vi "Logging Message Loop.vi"(8 "error in (no error)":errorcluster, 10 "Data Queue":T1, 11 "Message Queues":T2) -> (0 "error out":errorcluster)   [LabVIEW 2021, in "IMU Logging.lvlib"]
doc: "The message loop subVI to handle messages pertaining to logging data."
uses:
  IMU Logging.lvlib
  support/Message Queue/All Message Queues.ctl
  support/Message Queue/Message Cluster.ctl
  Acquisition/IMU Data Queue.ctl
  IMU TimeDataStruct.ctl
  Logging Configuration.ctl
  Logging State.ctl
  support/Message Queue/Enqueue Message (Single).vi
  <vilib>/Utility/error.llb/Error Cluster From Error Code.vi
  <vilib>/ErrorRing/Error Ring.xnode
  support/Message Queue/IMU Message Queue.lvlib
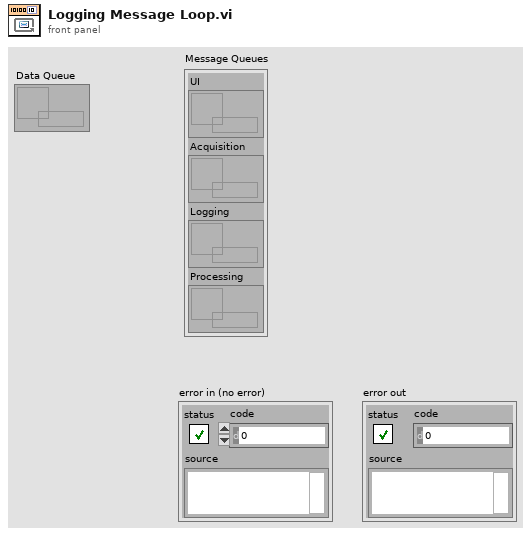
[diagram p1: front panel]
types:
  T1 = typedef "IMU Data Queue.ctl" = refnum<queue>
  T2 = typedef "IMU Message Queue.lvlib/All Message Queues.ctl" = cluster{"UI":refnum<queue>, "Acquisition":refnum<queue>, "Logging":refnum<queue>, "Processing":refnum<queue>}
  T3 = typedef "IMU Logging.lvlib/Logging Configuration.ctl" = cluster{"Log File Base Path":path, "TDMS File Reference":refnum<k34>, "Log Select":bool}
  T4 = typedef "IMU Logging.lvlib/Logging State.ctl" = enum16{"Idle", "Logging Turned off", "Logging"}
  T5 = enum16{"open", "open or create", "create or replace", "create", "open (read-only)"}
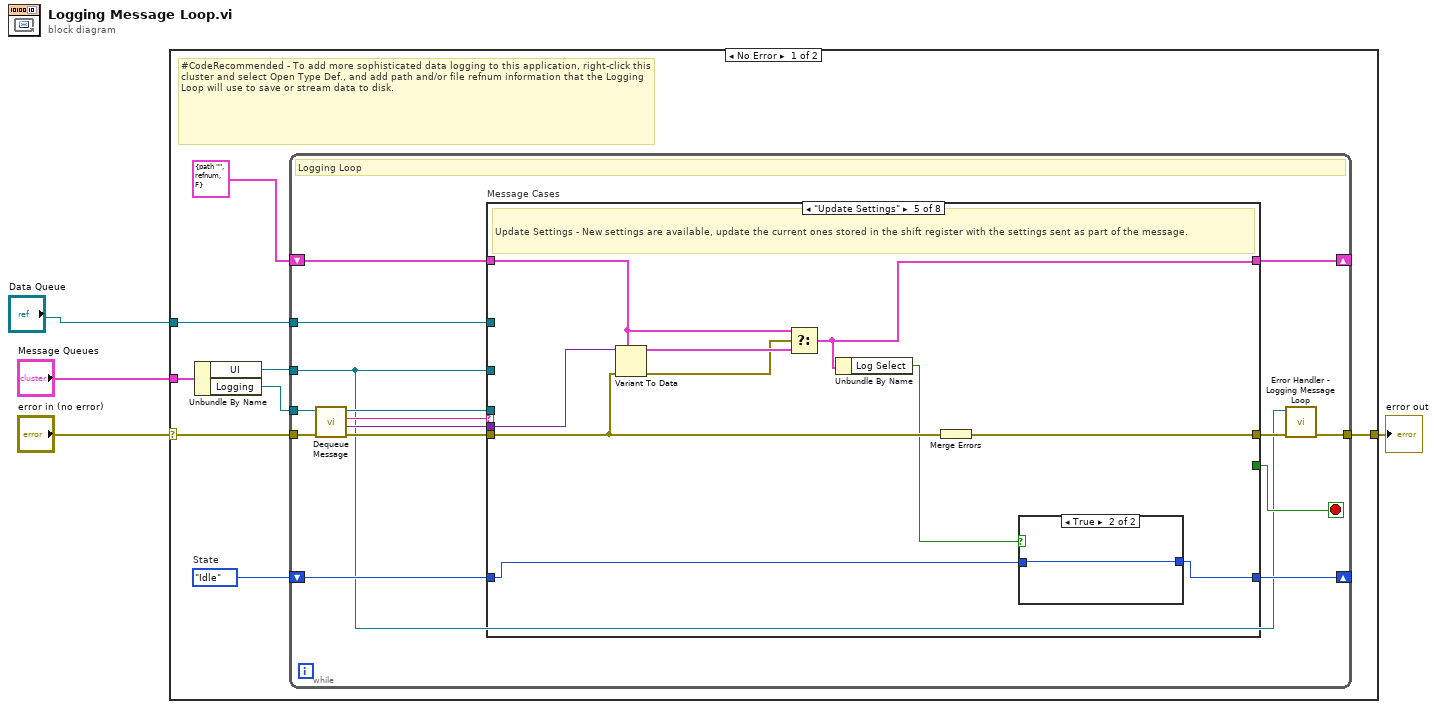
[diagram p0: block diagram]
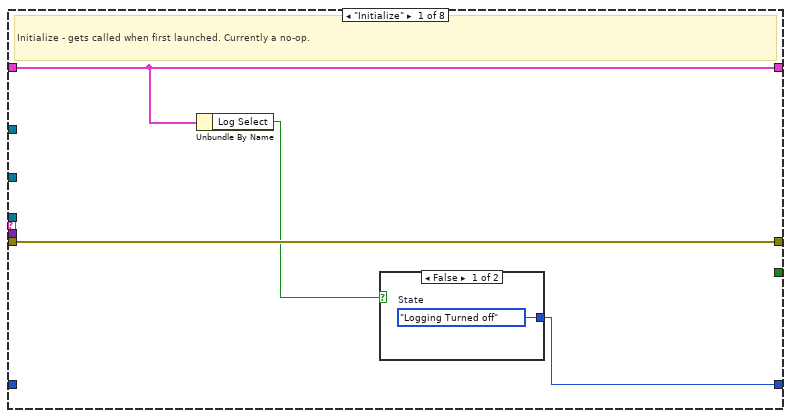
[diagram p2: hidden frame]
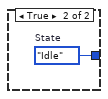
[diagram p3: hidden frame]
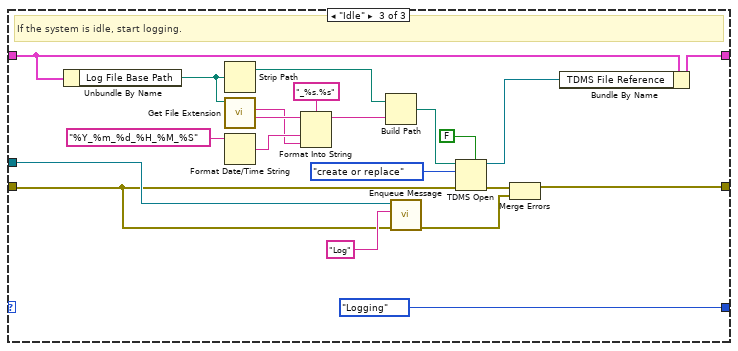
[diagram p6: hidden frame]
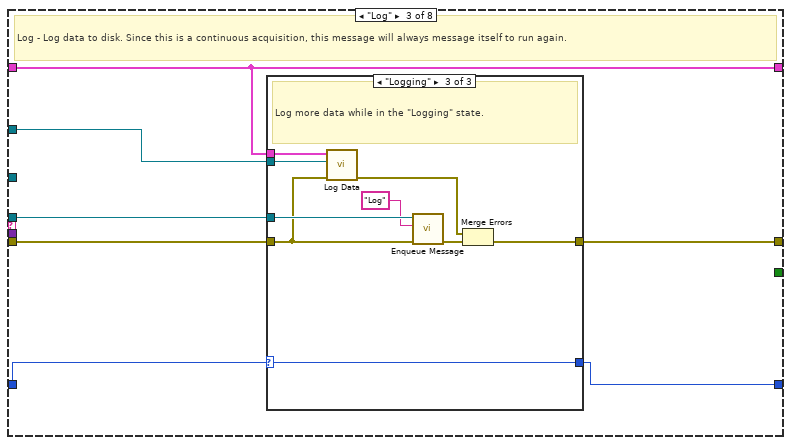
[diagram p7: hidden frame]
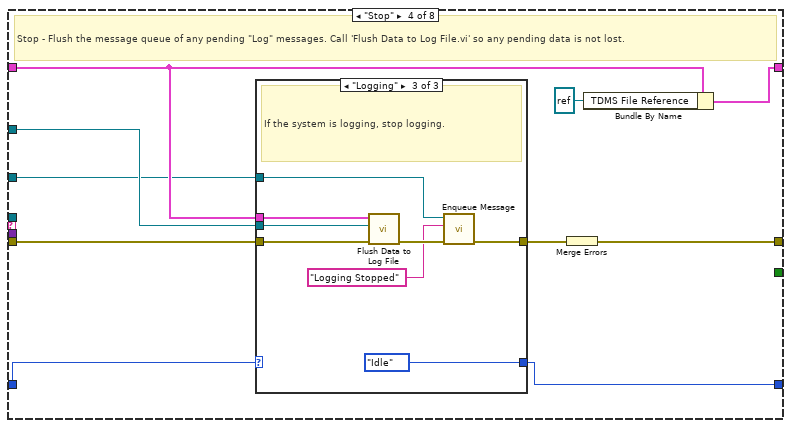
[diagram p10: hidden frame]
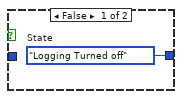
[diagram p13: hidden frame]
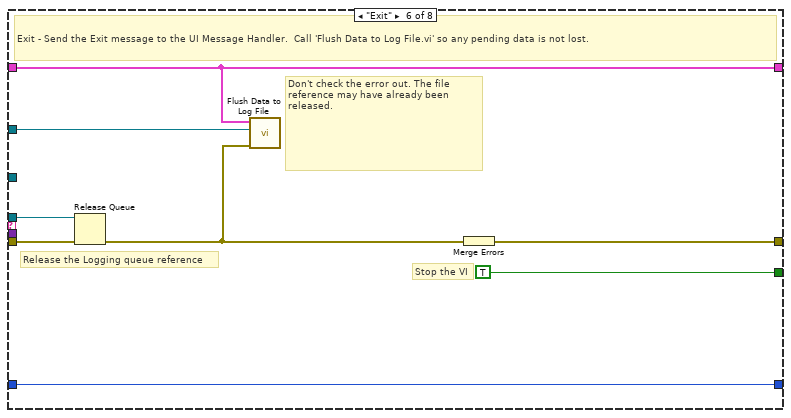
[diagram p14: hidden frame]
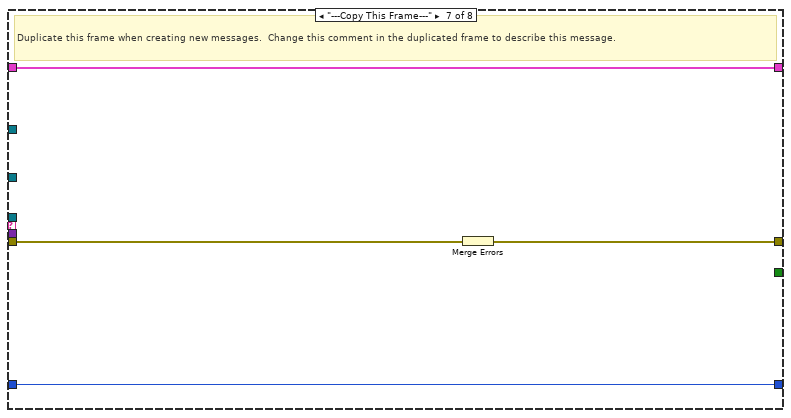
[diagram p15: hidden frame]
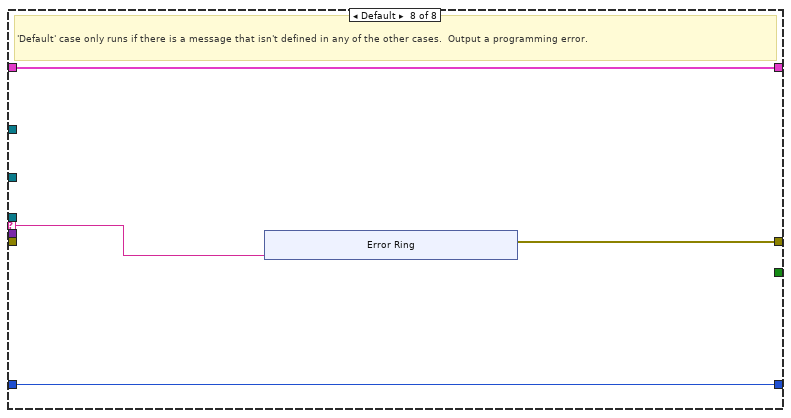
[diagram p16: hidden frame]
diagram:
  n1 = case shown="No Error" "error in (no error)" {
    selector: "error in (no error)" -> [w8 w145]
    tunnel: "Message Queues" -> [w12 _]
    tunnel: [w10 w145] -> w3
    tunnel: "Data Queue" -> [w7 _]
    frame No Error {
      w5 = Logging_State."Idle"  # State
      # "#CodeRecommended - To add more sophisticated data logging to this application, right-click this cluster and select Open Type Def., and add path and/or file refnum information that the Logging Loop will use to save or stream data to disk."
      n2 = Unbundle By Name(w12) -> ("UI"=w6:refnum<queue>, "Logging"=w11:refnum<queue>)
      n3 = while {
        tunnel: w11 -> [w19]
        shift-right: [w26] -> _
        shift-left: T3 {"Log File Base Path"=path "", "TDMS File Reference"=refnum, "Log Select"=FALSE} ("Logging Configuration") -> [w27]
        tunnel: w6 -> [w13]
        tunnel: w7 -> [w18]
        shift-right: [w16] -> _
        shift-left: w5 -> [w17]
        tunnel: w8 -> [w24]
        tunnel: [w15] -> w10
        stop <- w25 stop-if-true
        # "Logging Loop"
        n4 = call "Dequeue Message.vi"("error in (no error)"=w24, "Message Queue"=w19) -> ("error out"=w23:errorcluster, "Message Data"=w21:variant, "Message"=w22:string, "dup Message Queue"=w20:refnum<queue>)  [unwired: 6 in]
        n5 = case "Message Cases" shown="\"Update Settings\"" w22 {
          selector: w22 -> [_ _ _ _ _ _ _ w134]
          tunnel: w20 -> [_ w39 w73 _ _ w126 _ _]
          tunnel: w23 -> [w31 w38 w71 w91 w114 w127 w133 _]
          tunnel: [w31 w40 w74 w97 w119 w128 w131 w135] -> w14
          tunnel: w27 -> [w30 w37 w70 w92 w117 w124 w132 w137]
          tunnel: [w30 w36 w70 w95 w112 w124 w132 w137] -> w26
          tunnel: [_ _ _ _ _ TRUE _ _] -> w25
          tunnel: w21 -> [_ _ _ _ w118 _ _ _]
          tunnel: w13 -> [_ _ _ w88 _ _ _ _]
          tunnel: w18 -> [_ _ w72 w93 _ w123 _ _]
          tunnel: w17 -> [_ w35 w69 w90 w111 w122 w130 w136]
          tunnel: [w28 w34 w68 w89 w110 w122 w130 w136] -> w16
          frame "Initialize" {
            # "Initialize - gets called when first launched. Currently a no-op."
            n6 = Unbundle By Name(w30) -> ("Log Select"=w29:bool)
            n7 = case shown="False" w29 {
              tunnel: [w32 w33] -> w28
              frame False {
                w32 = Logging_State."Logging Turned off"  # State
              }
              frame True {
                w33 = Logging_State."Idle"  # State
              }
            }
          }
          frame "Start" {
            # "Start - Send the \"Log\" message to start logging.  Generate a unique, timestamped TDMS file name based on the Log File Base Path value."
            n8 = case shown="\"Logging Turned off\"" w35 {
              selector: w35 -> [w42 w45 _]
              tunnel: [w41 w44 w49] -> w40
              tunnel: w39 -> [_ _ w50]
              tunnel: w38 -> [w41 w44 w48]
              tunnel: w37 -> [w43 w46 w51]
              tunnel: [w43 w46 w53] -> w36
              tunnel: [w42 w45 Logging_State."Logging" ("State")] -> w34
              frame "Logging" {
                # "The system is already logging. Ignore the \"Start\" message."
              }
              frame "Logging Turned off" {
                # "The system is already logging. Ignore the \"Start\" message."
              }
              frame "Idle" {
                # "If the system is idle, start logging."
                n9 = Unbundle By Name(w51) -> ("Log File Base Path"=w66:path)
                n10 = Strip Path(path=w66) -> (stripped path=w63:path)  [unwired: 1 out]
                n11 = call <vilib>:"Get File Extension.vi"("file"=w66) -> ("filename without extension"=w64:string, "lowercase file extension"=w60:string)  [unwired: 6 in, 3 out]
                n12 = Format Date/Time String(time format string (%c)="%Y_%m_%d_%H_%M_%S") -> (date/time string=w61:string)  [unwired: 2 in]
                n13 = Format Into String(format string="_%s.%s", initial string=w64, w61, w60) -> (resulting string=w59:string)  [unwired: 1 in, 1 out]
                n14 = Build Path(base path=w63, name or relative path=w59) -> (appended path=w58:path)
                n15 = call-poly "Enqueue Message.vi"("error in (no error)"=w48, "Message"="Log", "Message Queue"=w50) -> ("error out"=w56:errorcluster)  [unwired: 7 in, 1 out]
                n16 = TDMS Open(5:FALSE ("create index file? (T)"), 8:w48, 10:T5."create or replace" ("operation (0:open)"), 11:w58) -> (0:w57:errorcluster, 3:w54:refnum<k34>)  [unwired: 3 in]
                n17 = Merge Errors(w57, w56) -> (w49:errorcluster)
                n18 = Bundle By Name(cluster=w51, "TDMS File Reference"=w54) -> (w53:T3)
              }
            }
          }
          frame "Log" {
            # "Log - Log data to disk. Since this is a continuous acquisition, this message will always message itself to run again."
            n19 = case shown="\"Logging\"" w69 {
              selector: w69 -> [w76 w78 w80]
              tunnel: [w75 w77 w87] -> w74
              tunnel: w73 -> [_ _ w85]
              tunnel: w72 -> [_ _ w84]
              tunnel: w71 -> [w75 w77 w79]
              tunnel: w70 -> [_ _ w81]
              tunnel: [w76 w78 w80] -> w68
              frame "Idle" {
                # "Ignore \"Log\" messages when the logging is idle."
              }
              frame "Logging Turned off" {
                # "Ignore \"Log\" messages when the logging is idle."
              }
              frame "Logging" {
                # "Log more data while in the \"Logging\" state."
                n20 = call "Log Data.vi"("error in (no error)"=w79, "Data Queue"=w84, "Logging Configuration"=w81) -> ("error out"=w83:errorcluster)  [unwired: 8 in]
                n21 = call-poly "Enqueue Message.vi"("error in (no error)"=w79, "Message"="Log", "Message Queue"=w85) -> ("error out"=w86:errorcluster)  [unwired: 7 in, 1 out]
                n22 = Merge Errors(w83, w86) -> (w87:errorcluster)
              }
            }
          }
          frame "Stop" {
            # "Stop - Flush the message queue of any pending \"Log\" messages. Call 'Flush Data to Log File.vi' so any pending data is not lost."
            n23 = case shown="\"Logging\"" w90 {
              selector: w90 -> [w98 w100 _]
              tunnel: [w99 w101 w104] -> w96
              tunnel: w93 -> [_ _ w108]
              tunnel: w92 -> [_ _ w107]
              tunnel: w91 -> [w99 w101 w106]
              tunnel: [w98 w100 Logging_State."Idle" ("State")] -> w89
              tunnel: w88 -> [_ _ w103]
              frame "Idle" {
                # "The system is already idle. Ignore the \"Stop\" message."
              }
              frame "Logging Turned off" {
                # "The system is already idle. Ignore the \"Stop\" message."
              }
              frame "Logging" {
                # "If the system is logging, stop logging."
                n24 = call "Flush Data to Log File.vi"("error in (no error)"=w106, "Data Queue"=w108, "Logging Configuration"=w107) -> ("error out"=w109:errorcluster)  [unwired: 8 in]
                n25 = call-poly "Enqueue Message.vi"("error in (no error)"=w109, "Message"="Logging Stopped", "Message Queue"=w103) -> ("error out"=w104:errorcluster)  [unwired: 7 in, 1 out]
              }
            }
            n26 = Merge Errors(w96) -> (w97:errorcluster)
            n27 = Bundle By Name(cluster=w92, "TDMS File Reference"=refnum<k34> refnum) -> (w95:T3)
          }
          frame "Update Settings" {
            # "Update Settings - New settings are available, update the current ones stored in the shift register with the settings sent as part of the message."
            n28 = Variant To Data(error in=w114, type=w117, Variant=w118) -> (data=w116:T3, error out=w115:errorcluster)
            n29 = Select(t=w117, s=w115, f=w116) -> (s? t:f=w112:T3)
            n30 = Unbundle By Name(w112) -> ("Log Select"=w113:bool)
            n31 = Merge Errors(w114) -> (w119:errorcluster)
            n32 = case shown="True" w113 {
              tunnel: [w120 w121] -> w110
              tunnel: w111 -> [_ w121]
              frame False {
                w120 = Logging_State."Logging Turned off"  # State
              }
              frame True {
              }
            }
          }
          frame "Exit" {
            # "Don't check the error out. The file reference may have already been released."
            # "Release the Logging queue reference"
            # "Stop the VI"
            # "Exit - Send the Exit message to the UI Message Handler.  Call 'Flush Data to Log File.vi' so any pending data is not lost."
            n33 = Release Queue(queue=w126, error in (no error)=w127) -> (error out=w125:errorcluster)  [unwired: 1 in, 2 out]
            n34 = call "Flush Data to Log File.vi"("error in (no error)"=w125, "Data Queue"=w123, "Logging Configuration"=w124) -> ()  [unwired: 8 in, 1 out]
            n35 = Merge Errors(w125) -> (w128:errorcluster)
          }
          frame "---Copy This Frame---" {
            # "Duplicate this frame when creating new messages.  Change this comment in the duplicated frame to describe this message."
            n36 = Merge Errors(w133) -> (w131:errorcluster)
          }
          frame Default {
            # "'Default' case only runs if there is a message that isn't defined in any of the other cases.  Output a programming error."
            n37 = xnode "Error Ring"("parameter 0"=w134) -> ("error out"=w135:errorcluster)
          }
        }
        n38 = call "Error Handler - Logging Message Loop.vi"("error in (no error)"=w14, "Message Queue"=w13) -> ("dup error in"=w15:errorcluster)  [unwired: 8 in, 1 out]
      }
    }
    frame Error {
    }
  }
  "error out" <- w3
